vi "Convert GP354 Pressure.vi"(1 "Input Byte 2":u8, 2 "Input Byte 1":u8) -> (0 "Pressure":dbl)   [LabVIEW 2011]
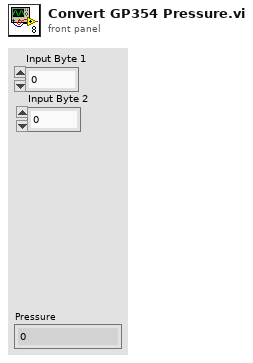
[diagram p1: front panel]
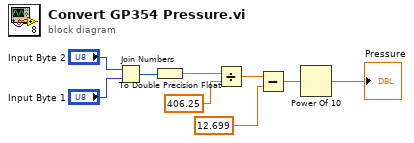
[diagram p0: block diagram]
diagram:
  n1 = Join Numbers(hi="Input Byte 2", lo="Input Byte 1") -> ((hi.lo)=w1:u16)
  n2 = To Double Precision Float(number=w1) -> (double precision float=w5:dbl)
  n3 = Divide(x=w5, y=406.25) -> (x/y=w8:dbl)
  n4 = Subtract(x=w8, y=12.699) -> (x-y=w6:dbl)
  n5 = Power Of 10(x=w6) -> (10^x=→"Pressure":dbl)
